vi "applyInsertSpaceX.vi"(6 "deltaX":u16, 8 "error in (no error)":errorcluster, 10 "originX":i32, 11 "Structure in":refnum<class "Structure.lvclass">) -> (0 "error out":errorcluster, 3 "Structure out":refnum<class "Structure.lvclass">)   [LabVIEW 2023, in "TLC_Scripto.lvlib" / "Structure.lvclass"]
uses:
  Structure.lvclass
  Structure.lvclass/Structure.ctl
  AbstractDiagram/AbstractDiagram.lvclass
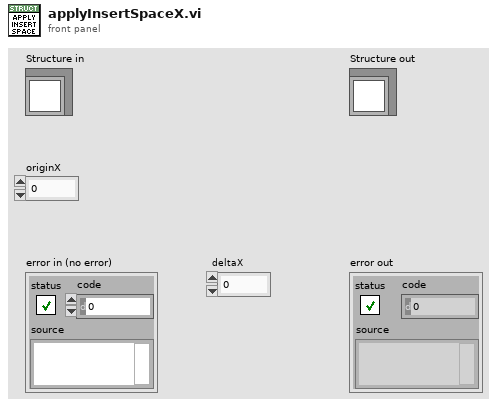
[diagram p1: front panel]
types:
  T1 = typedef "TLC_Scripto.lvlib/rectangle.ctl" = cluster{"left":i32, "top":i32, "right":i32, "bottom":i32}
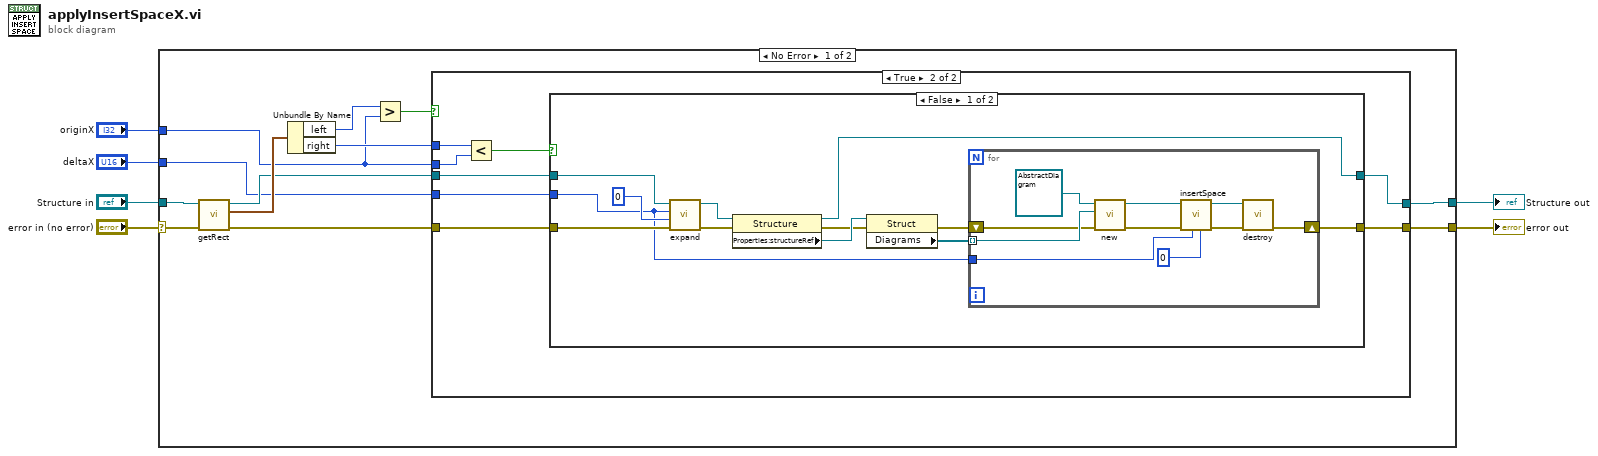
[diagram p0: block diagram]
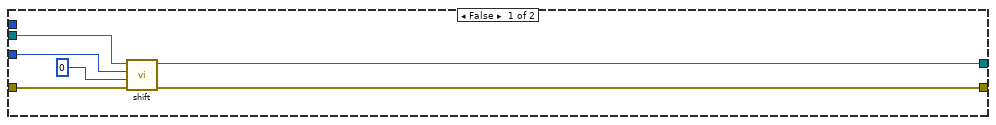
[diagram p2: hidden frame]
diagram:
  n1 = case shown="No Error" "error in (no error)" {
    selector: "error in (no error)" -> [w18 w58]
    tunnel: [w12 w58] -> w6
    tunnel: [w10 w57] -> w5
    tunnel: "deltaX" -> [w9 _]
    tunnel: "originX" -> [w7 _]
    tunnel: "Structure in" -> [w16 w57]
    frame No Error {
      n2 = call-dynamic "getRect.vi"("error in (no error)"=w18, "GObject in"=w16) -> ("error out"=w13:errorcluster, "rectangle"=w17:T1, "GObject out"=w11:refnum<class "Structure.lvclass">)  [unwired: 7 in]
      n3 = Unbundle By Name(w17) -> ("left"=w15:i32, "right"=w8:i32)
      n4 = Greater?(x=w15, y=w7) -> (0:w14:bool)
      n5 = case shown="True" w14 {
        tunnel: w13 -> [w22 w29]
        tunnel: [w21 w28] -> w12
        tunnel: w11 -> [w24 w27]
        tunnel: [w23 w26] -> w10
        tunnel: w9 -> [w20 w25]
        tunnel: w8 -> [_ w32]
        tunnel: w7 -> [_ w31]
        frame False {
          n6 = call-dynamic "shift.vi"("error in (no error)"=w22, "deltaY[pixel]"=0, "deltaX[pixel]"=w20, "GObject in"=w24) -> ("error out"=w21:errorcluster, "GObject out"=w23:refnum<class "Structure.lvclass">)  [unwired: 6 in]
        }
        frame True {
          n7 = Less?(x=w32, y=w31) -> (x < y?=w30:bool)
          n8 = case shown="False" w30 {
            tunnel: [w34 w56] -> w28
            tunnel: w29 -> [w43 w56]
            tunnel: w27 -> [w44 w55]
            tunnel: [w39 w55] -> w26
            tunnel: w25 -> [w33 _]
            frame False {
              n9 = call "expand.vi"("error in (no error)"=w43, "expansion_y"=u32 0, "expansion_x"=w33, "Structure in"=w44) -> ("error out"=w41:errorcluster, "Structure out"=w40:refnum<class "Structure.lvclass">)  [unwired: 6 in]
              n10 = property class="Structure"(reference=w40, error in=w41) -> (reference out=w39:refnum<class "Structure.lvclass">, error out=w37:errorcluster, "Properties:structureRef"=w38:refnum<vi>)
              n11 = property class="Struct"(reference=w38, error in=w37) -> (error out=w35:errorcluster, "Diagrams"=w36:refnum<vi>[])  [unwired: 1 out]
              n12 = for {
                tunnel: w36 -> [w53] mode=indexing
                shift-right: [w48] -> w34
                shift-left: w35 -> [w52]
                tunnel: w33 -> [w45]
                n13 = call-dynamic "new.vi"("Error In"=w52, "ref"=w53, "Generic In"=refnum<class "AbstractDiagram.lvclass"> refnum ("TLC_Scripto.lvlib:AbstractDiagram.lvclass")) -> ("Error Out"=w50:errorcluster, "Generic Out"=w51:refnum<class "AbstractDiagram.lvclass">)  [unwired: 7 in]
                n14 = call "insertSpace.vi"("deltaY"=u16 0, "deltaX"=w45, "error in (no error)"=w50, "BlockDiagram in"=w51) -> ("error out"=w49:errorcluster, "BlockDiagram out"=w47:refnum<class "AbstractDiagram.lvclass">)  [unwired: 6 in]
                n15 = call-dynamic "destroy.vi"("Error In"=w49, "Generic In"=w47) -> ("Error Out"=w48:errorcluster)  [unwired: 9 in]
              }
            }
            frame True {
              # "Nothing to do"
            }
          }
        }
      }
    }
    frame Error {
    }
  }
  "error out" <- w6
  "Structure out" <- w5
